vi "前站查询.vi"(10 "DBSet":T1, 11 "SN":string) -> (3 "判定":bool)   [LabVIEW 2011]
panel:
  out "维修OK":bool
  out "不良存在":bool
  out "id":string
  out "查询数据":string[][](array[string])
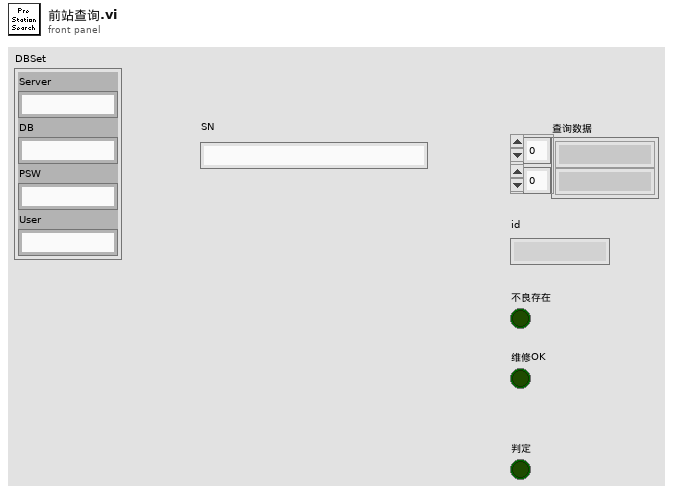
[diagram p1: front panel]
types:
  T1 = cluster{"Server":string, "DB":string, "PSW":string, "User":string}
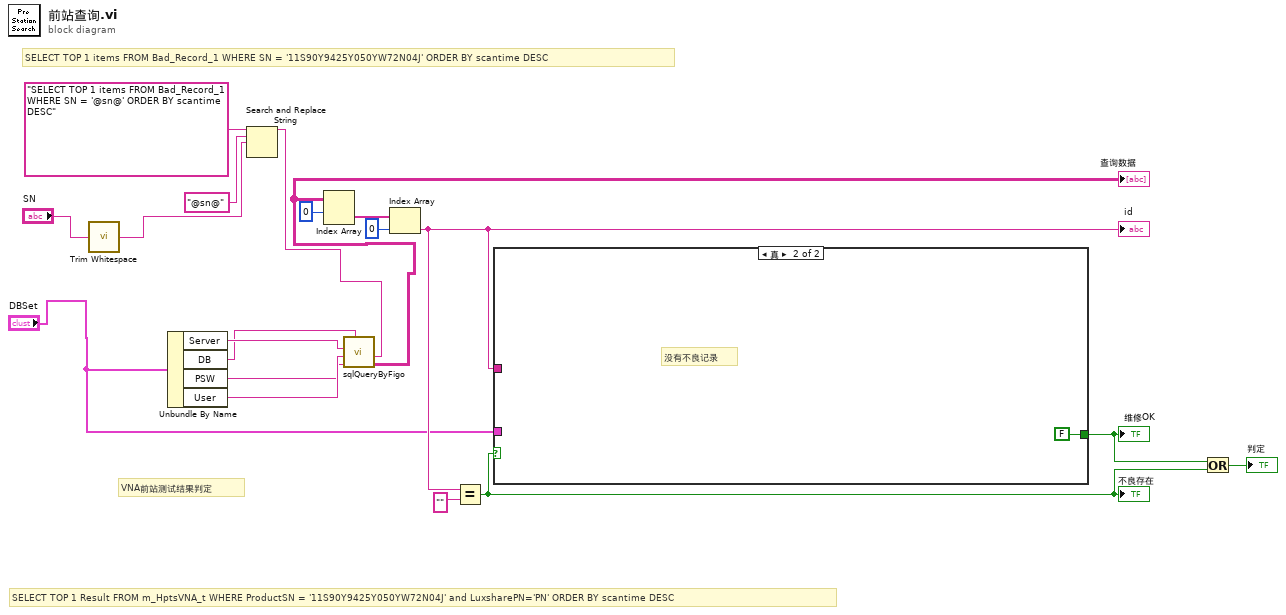
[diagram p0: block diagram]
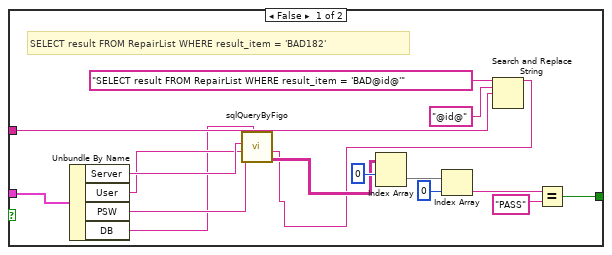
[diagram p2: hidden frame]
diagram:
  # "SELECT TOP 1 Result FROM m_HptsVNA_t WHERE ProductSN = '11S90Y9425Y050YW72N04J' and LuxsharePN='PN' ORDER BY scantime DESC"
  # "VNA前站测试结果判定"
  # "SELECT TOP 1 items FROM Bad_Record_1 WHERE SN = '11S90Y9425Y050YW72N04J' ORDER BY scantime DESC"
  n1 = call <vilib>:"Trim Whitespace.vi"("string"="SN") -> ("trimmed string"=w8:string)  [unwired: 1 in]
  n2 = Unbundle By Name("DBSet") -> ("Server"=w4:string, "DB"=w1:string, "PSW"=w2:string, "User"=w3:string)
  n3 = Search and Replace String(input string="SELECT TOP 1 items FROM Bad_Record_1 WHERE SN = '@sn@' ORDER BY scantime DESC", search string="@sn@" ("搜索字符串"), replace string=w8) -> (result string=w5:string)  [unwired: 5 in, 3 out]
  n4 = call "sqlQueryByFigo.vi"("SQL"=w5, "DATABASE"=w1, "password"=w2, "user id"=w3, "Server"=w4) -> ("查询数据"=w6:string[][])  [unwired: 5 in, 1 out]
  "查询数据" <- w6
  n5 = Index Array(array=w6, index (row)=0 ("索引 (行)")) -> (element=w16:string[])  [unwired: 1 in]
  n6 = Index Array(array=w16, index=0 ("索引")) -> (element=w13:string)
  "id" <- w13
  n7 = Equal?(x=w13, y="") -> (x = y?=w11:bool)
  "不良存在" <- w11
  n8 = case shown="真" w11 {
    tunnel: w13 -> [w33 _]
    tunnel: [w27 FALSE] -> w12
    tunnel: "DBSet" -> [w24 _]
    frame False {
      # "SELECT result FROM RepairList WHERE result_item = 'BAD182'"
      n9 = Unbundle By Name(w24) -> ("Server"=w23:string, "User"=w22:string, "PSW"=w21:string, "DB"=w20:string)
      n10 = Search and Replace String(input string="SELECT result FROM RepairList WHERE result_item = 'BAD@id@'", search string="@id@" ("搜索字符串"), replace string=w33) -> (result string=w25:string)  [unwired: 5 in, 3 out]
      n11 = call "sqlQueryByFigo.vi"("SQL"=w25, "DATABASE"=w20, "password"=w21, "user id"=w22, "Server"=w23) -> ("查询数据"=w26:string[][])  [unwired: 5 in, 1 out]
      n12 = Index Array(array=w26, index (row)=0 ("索引 (行)")) -> (element=w31:string[])  [unwired: 1 in]
      n13 = Index Array(array=w31, index=0 ("索引")) -> (element=w29:string)
      n14 = Equal?(x=w29, y="PASS") -> (x = y?=w27:bool)
    }
    frame True {
      # "没有不良记录"
    }
  }
  "维修OK" <- w12
  n15 = Or(x=w12, y=w11) -> (x .or. y?=→"判定":bool)
